vi "Set Defaults.vi"(11 "Long Class Name Entity Example in":refnum<class "Long Class Name Entity Example.lvclass">) -> (3 "Long Class Name Entity Example out":refnum<class "Long Class Name Entity Example.lvclass">)   [LabVIEW 2022 SP3, in "Conditum-Example.lvlib" / "Long Class Name Entity Example.lvclass"]
uses:
  Long Class Name Entity Example.lvclass
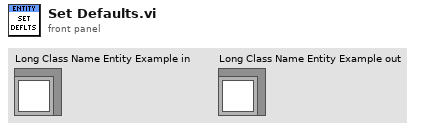
[diagram p1: front panel]
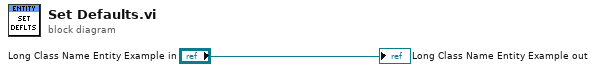
[diagram p0: block diagram]
diagram:
  "Long Class Name Entity Example out" <- "Long Class Name Entity Example in"
